vi "IPI——Signal Test.vi"() -> ()   [LabVIEW 2015]
panel:
  out "数值":i32
  out "数组 2":string[](array[string])
  out "All Files in Dir":path[](array[path]) caption="目录中的所有文件"
  out "数组":string[](array[string])
  out "Distance piexl":string
  in  "File Path":path=path "C:/GapAndFlatnessMesaure/Source Code/Image/AutoRun-Step3-CCD-Snap1.bmp"
  out "Distance mm":string
  out "Image":T1(plugin-control)
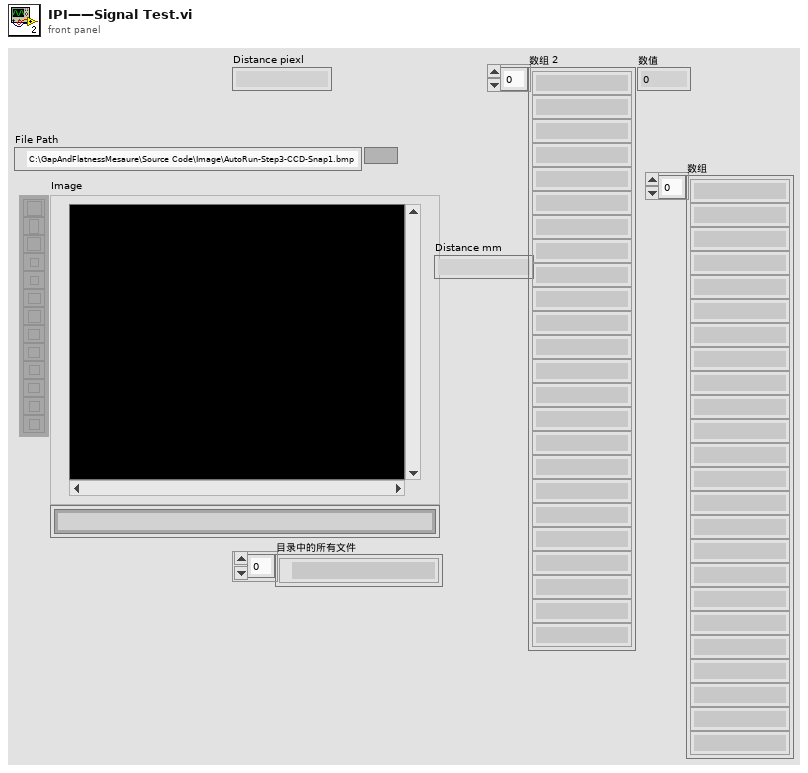
[diagram p1: front panel]
types:
  T1 = typedef "IMAQ Image.ctl" = refnum<image>
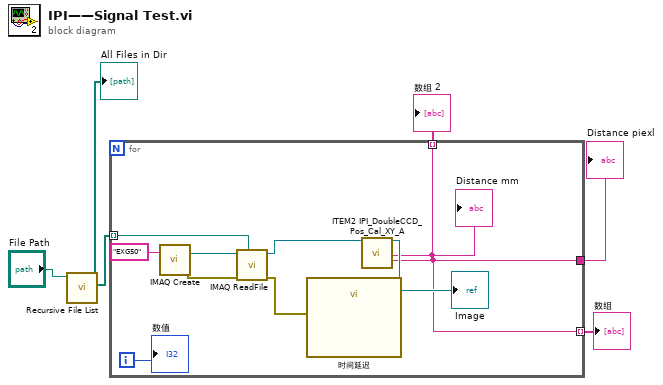
[diagram p0: block diagram]
diagram:
  n1 = call <vilib>:"Recursive File List.vi"("Folder Path"="File Path") -> ("All Files in Dir"=w3:path[])  [unwired: 6 in, 4 out]
  "All Files in Dir" <- w3
  n2 = for {
    tunnel: [w9] -> w5
    tunnel: w3 -> [w10] mode=indexing
    tunnel: [w9] -> w2 mode=indexing
    tunnel: [w8] -> w1 mode=indexing
    i -> [w6]
    n3 = call "IMAQ Create"("Image Name"="EXG50") -> ("New Image"=w13:T1, "error out"=w15:errorcluster)  [unwired: 4 in]
    n4 = call "IMAQ ReadFile"("File Path"=w10, "error in (no error)"=w15, "Image"=w13) -> ("error out"=w7:errorcluster, "Image Out"=w12:T1)  [unwired: 4 in, 3 out]
    n5 = call "时间延迟"("error in (no error)"=w7) -> ()  [unwired: 10 in, 1 out]
    n6 = call "ITEM2 IPI_DoubleCCD_Pos_Cal_XY_A.vi"("Image In"=w12) -> ("Image"=→"Image":T1, "Distance mm"=w8:string, "Distance piexl"=w9:string)  [unwired: 13 in, 3 out]
    "Distance mm" <- w8
    "数值" <- w6
  }
  "Distance piexl" <- w5
  "数组" <- w2
  "数组 2" <- w1
